vi "CheckOutput.vi"(8 "Target Binary Output":bool[](array[boolean]), 9 "Actual Binary Output":bool[](array[boolean]), 11 "Expected Output Pin":i32) -> (1 "Pin to Train":i32, 2 "logical AND":bool)   [LabVIEW 2018]
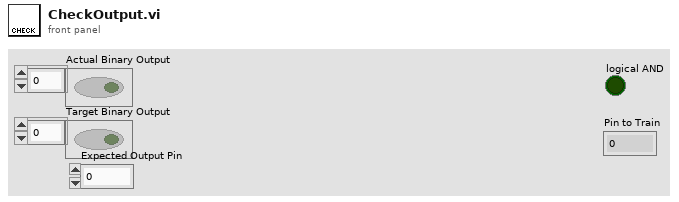
[diagram p1: front panel]
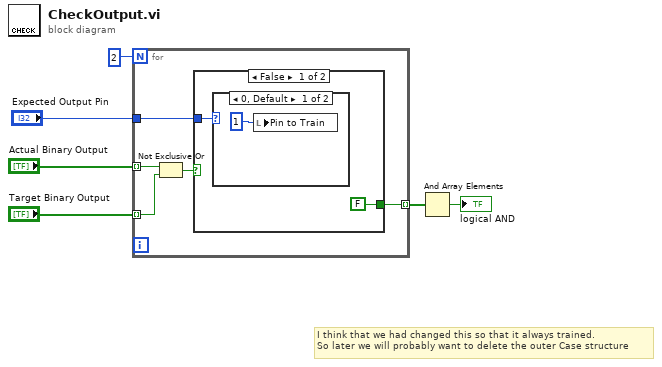
[diagram p0: block diagram]
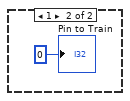
[diagram p2: hidden frame]
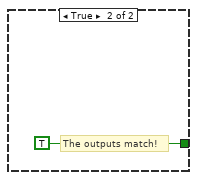
[diagram p3: hidden frame]
diagram:
  # "I think that we had changed this so that it always trained.\nSo later we will probably want to delete the outer Case structure"
  n1 = for {
    N: 2 -> [_]
    tunnel: [w10] -> w3 mode=indexing
    tunnel: "Actual Binary Output" -> [w9] mode=indexing
    tunnel: "Target Binary Output" -> [w8] mode=indexing
    tunnel: "Expected Output Pin" -> [w7]
    n2 = Not Exclusive Or(1:w8, 2:w9) -> (0:w11:bool)
    n3 = case shown="False" w11 {
      tunnel: [FALSE ("Ouputs Match") TRUE] -> w10
      tunnel: w7 -> [w12 _]
      frame False {
        n4 = case shown="0, Default" w12 {
          frame 0, Default {
            n5 = local write "Pin to Train"(1 ("Pin To Train 2")) -> ()
          }
          frame 1 {
            "Pin to Train" <- 0 ("Pin to Train")
          }
        }
      }
      frame True {
        # "The outputs match!"
      }
    }
  }
  n6 = And Array Elements(Boolean array=w3) -> (logical AND=→"logical AND":bool)
